vi "Removedor de outliers.vi"(1 "Vetor de tensão in":dbl[](array[numeric])) -> (0 "Média":dbl)   [LabVIEW 2013]
uses:
  <vilib>/Analysis/NI_AALBase.lvlib
  <vilib>/Analysis/baseanly.llb/Mean (DBL).vi
panel:
  in  "Voltar":bool
  out "Desvio padrão":dbl
  out "Média":dbl
  in  "Cortar":bool
  in  "Pronto":bool
  out "Dados":waveform(dbl)(graph)
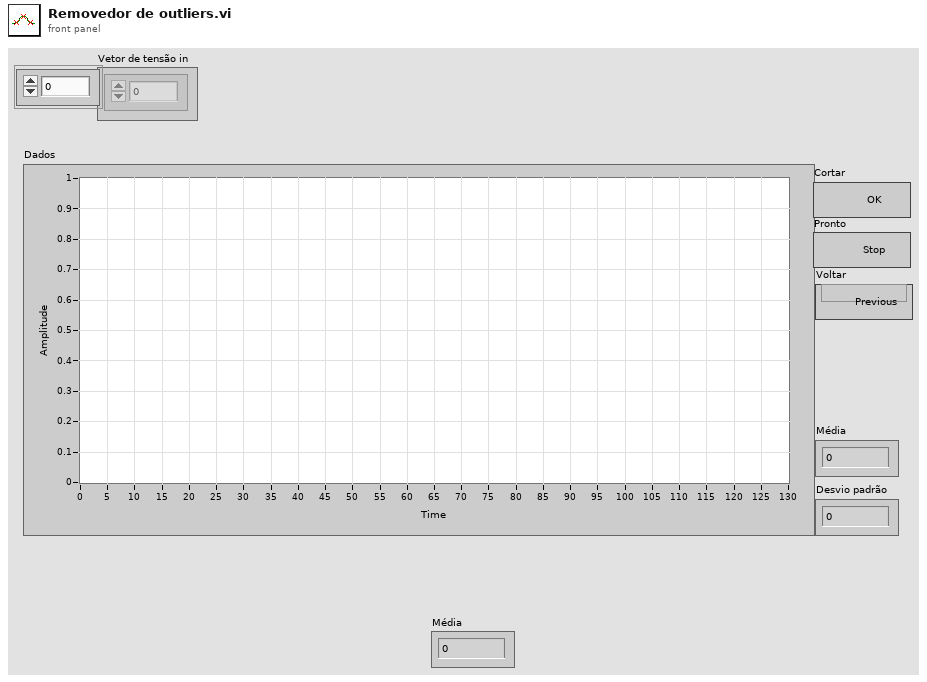
[diagram p1: front panel]
types:
  T1 = typedef "LVCursorListTypeDef.ctl" = cluster{"Name":string, "Color":u32, "Style":u8, "Point Style":u8, "Name Visible":bool, "Allow Drag":bool, "Cursor Mode":u32, "Plot":i32, "Index":i32, "Position":cluster{"X":dbl, "Y":dbl}, "X Scale":u32, "Y Scale":u32, "Watch Plots":i32[], "Watch All Plots":bool, "Plot Area":i32, "Label Offset":cluster{"X":dbl, "Y":dbl}}[]
  T2 = cluster{"Name":string, "Color":u32, "Style":u8, "Point Style":u8, "Name Visible":bool, "Allow Drag":bool, "Cursor Mode":u32, "Plot":i32, "Index":i32, "Position":cluster{"X":dbl, "Y":dbl}, "X Scale":u32, "Y Scale":u32, "Watch Plots":i32[], "Watch All Plots":bool, "Plot Area":i32, "Label Offset":cluster{"X":dbl, "Y":dbl}}
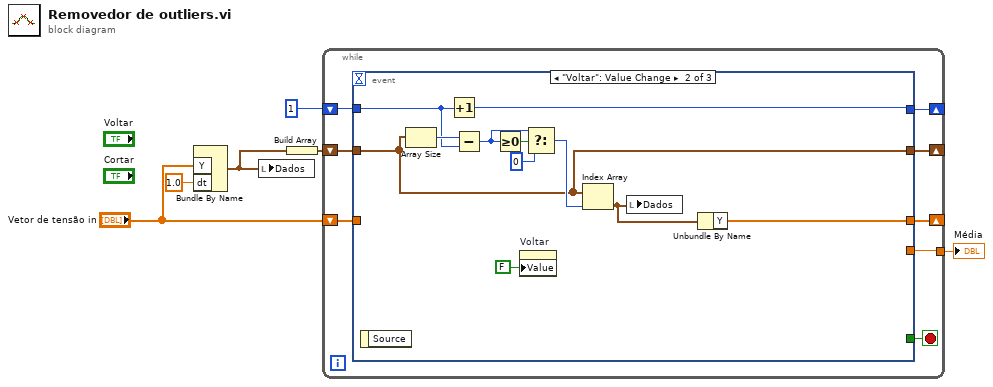
[diagram p0: block diagram]
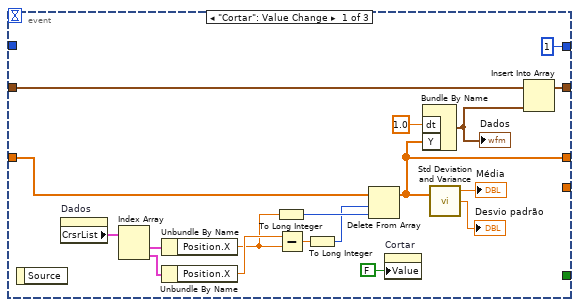
[diagram p2: hidden frame]
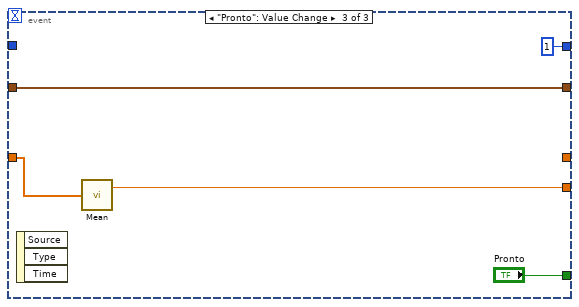
[diagram p3: hidden frame]
diagram:
  n1 = Bundle By Name("Y"="Vetor de tensão in", "dt"=1.0) -> (w4:waveform(dbl))  [unwired: 1 in]
  n2 = local write "Dados"(w4) -> ()
  n3 = Build Array(w4) -> (w3:waveform(dbl)[])
  n4 = while {
    shift-right: [w12] -> _
    shift-left: "Vetor de tensão in" -> [w11]
    tunnel: [w13] -> w6
    shift-right: [w9] -> _
    shift-left: w3 -> [w10]
    shift-right: [w7] -> _
    shift-left: 1 -> [w8]
    stop <- w14 stop-if-true
    n5 = event shown="[1] \"Voltar\": Value Change" {
      selector: _ -> [_ _ _]
      dyn-events: _ -> [_ _ _]
      timeout: _ -> [_ _ _]
      tunnel: w11 -> [w18 _ w47]
      tunnel: [_ _ "Pronto"] -> w14
      tunnel: [_ _ w46] -> w13
      tunnel: [w15 w33 _] -> w12
      tunnel: w10 -> [w20 w35 w44]
      tunnel: [w19 w35 w44] -> w9
      tunnel: w8 -> [_ w38 _]
      tunnel: [1 w37 1] -> w7
      event "Cortar": Value Change {
        n6 = event-data() -> ()  [unwired: 1 in, 1 out]
        n7 = property on="Dados" class="WFGraph (strict)"() -> ("CrsrList"=w32:T1)  [unwired: 2 in, 2 out]
        n8 = Index Array(array=w32) -> (element #1=w31:T2, element #2=w30:T2)  [unwired: 2 in]
        n9 = Unbundle By Name(w31) -> ("Position.X"=w27:dbl)
        n10 = Unbundle By Name(w30) -> ("Position.X"=w29:dbl)
        n11 = To Long Integer(number=w27) -> (32bit integer=w26:i32)
        n12 = Subtract(x=w29, y=w27) -> (x-y=w28:dbl)
        n13 = To Long Integer(number=w28) -> (32bit integer=w25:i32)
        n14 = Delete From Array(array=w18, length=w25, index=w26) -> (array with subset deleted=w15:dbl[])  [unwired: 1 out]
        n15 = property on="Cortar" class="Bool (strict)"("Value"=FALSE ("Cortar")) -> ()  [unwired: 2 in, 2 out]
        n16 = Bundle By Name("dt"=1.0, "Y"=w15) -> (w21:waveform(dbl))  [unwired: 1 in]
        "Dados" <- w21
        n17 = call <vilib>:"Std Deviation and Variance.vi"("X"=w15) -> ("mean"=→"Média":dbl, "standard deviation"=→"Desvio padrão":dbl)  [unwired: 1 in, 1 out]
        n18 = Insert Into Array(array=w20, new element=w21) -> (w19:waveform(dbl)[])  [unwired: 1 in]
      }
      event "Voltar": Value Change {
        n19 = event-data() -> ()  [unwired: 1 in, 1 out]
        n20 = Array Size(array=w35) -> (size(s)=w42:i32)
        n21 = Increment(x=w38) -> (x+1=w37:i32)
        n22 = Subtract(x=w42, y=w38) -> (x-y=w41:i32)
        n23 = Greater Or Equal To 0?(x=w41) -> (x >= 0?=w43:bool)
        n24 = property on="Voltar" class="Bool (strict)"("Value"=FALSE ("Voltar")) -> ()  [unwired: 2 in, 2 out]
        n25 = Select(t=w41, s=w43, f=0) -> (s? t:f=w39:i32)
        n26 = Index Array(array=w35, index=w39) -> (element=w34:waveform(dbl))
        n27 = local write "Dados"(w34) -> ()
        n28 = Unbundle By Name(w34) -> ("Y"=w33:dbl[])
      }
      event "Pronto": Value Change {
        n29 = event-data() -> ()  [unwired: 1 in, 3 out]
        n30 = call-poly <vilib>:"Mean.vi"("X"=w47) -> ("mean"=w46:dbl)  [unwired: 1 out]
      }
    }
  }
  "Média" <- w6
